vi "Atto DRY Interface get User Temperature.vi"(8 "error in (no error)":errorcluster, 11 "Temperature":sgl) -> (0 "error out":errorcluster, 2 "function return":i32, 3 "Temperature out":sgl)   [LabVIEW 2016, in "attoDRYLib.lvlib"]
doc: "int32_t __cdecl AttoDRY_Interface_getUserTemperature(float *Temperature);"
uses:
  <userlib>/attoDRYLib/attoDRYLib.lvlib
  <userlib>/attoDRYLib/attoDRYLib.dll
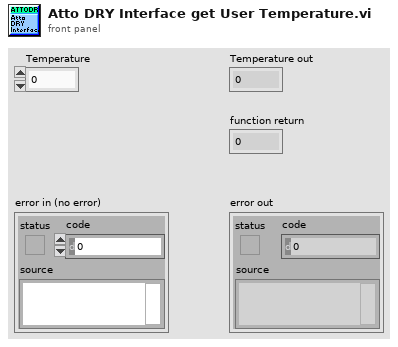
[diagram p1: front panel]
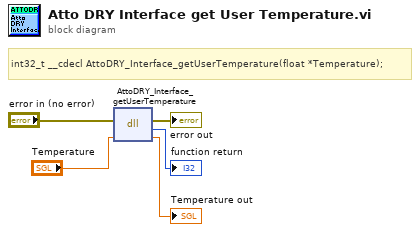
[diagram p0: block diagram]
diagram:
  # "int32_t __cdecl AttoDRY_Interface_getUserTemperature(float *Temperature);"
  n1 = dll-call lib="C:/Program Files (x86)/National Instruments/LabVIEW 2016/user.lib/attoDRYLib/attoDRYLib.*" fn="AttoDRY_Interface_getUserTemperature"(error in="error in (no error)", "Temperature"="Temperature") -> (error out=→"error out":errorcluster, →"function return":i32, "Temperature"=→"Temperature out":sgl)  [unwired: 2 in, 1 out]
